vi "Get Acquisition Data.vi"(4 "error in (no error)":errorcluster, 6 "Bytes to read (0)":u32 max=1000, 7 "VISA resource name":refnum<visa-resource-name>) -> (0 "error out":errorcluster, 2 "Data":i32[](array[numeric]) format="%.0x", 3 "VISA resource name out":refnum<visa-resource-name>)   [LabVIEW 2020, in "Newport ESP301.lvlib"]
doc: "This command is used to retrieve data acquired from a data acquisition request.\nThis command returns byte wide binary data. Each four bytes represents one DSP 32 bit word. The number of bytes returned depends on the setup request. (See DC command)."
uses:
  Newport ESP301.lvlib
panel:
  out "Data Acquired":string
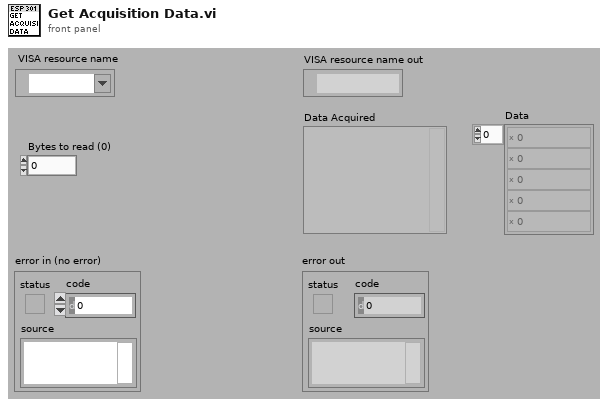
[diagram p1: front panel]
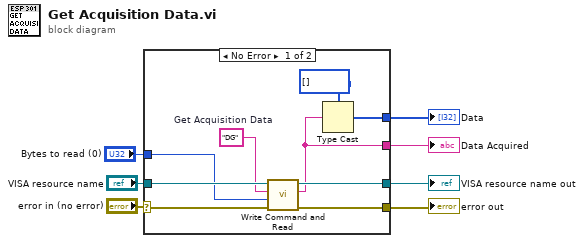
[diagram p0: block diagram]
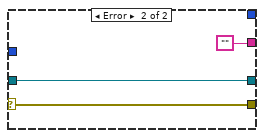
[diagram p2: hidden frame]
diagram:
  n1 = case shown="No Error" "error in (no error)" {
    selector: "error in (no error)" -> [w13 w19]
    tunnel: [w15 w19] -> w7
    tunnel: "VISA resource name" -> [w16 w18]
    tunnel: [w14 w18] -> w6
    tunnel: [w10 ""] -> w3
    tunnel: "Bytes to read (0)" -> [w11 _]
    tunnel: [w8 _] -> w1
    frame No Error {
      w12 = "DG"  # Get Acquisition Data
      n2 = call "Write Command and Read.vi"("error in (no error)"=w13, "Bytes to read (100)"=w11, "Command"=w12, "VISA resource name"=w16) -> ("error out"=w15:errorcluster, "Returned string"=w10:string, "VISA resource name out"=w14:refnum<visa-resource-name>)  [unwired: 3 in]
      n3 = Type Cast(type=i32[] [], x=w10) -> (*(type *) &x=w8:i32[])
    }
    frame Error {
    }
  }
  "error out" <- w7
  "VISA resource name out" <- w6
  "Data Acquired" <- w3
  "Data" <- w1
